vi "GE 5565PIORC.DMA.Block.In-Place Read (DBL).vi"(7 "count (-1: all)":i32=-1, 8 "error in (no error)":errorcluster, 9 "data in":dbl[](array[numeric]), 10 "Block Descriptor in":T1 {"descriptor params"."data ptr (lower)" format="%.0x"; "descriptor params"."data ptr (upper)" format="%.0x"; "descriptor params"."data size" format="%.0x"; "descriptor params"."next descriptor ptr" format="%.0x"; "descriptor size" format="%08x"; "descriptor ptr (RFM)" format="%08x"; "descriptor ptr (VISA)" format="%08x"}, 11 "GE 5565PIORC in":refnum<class "GE 5565PIORC.lvclass">) -> (0 "error out":errorcluster, 1 "data out":dbl[](array[numeric]), 2 "Block Descriptor out":T1 {"descriptor params"."data ptr (lower)" format="%.0x"; "descriptor params"."data ptr (upper)" format="%.0x"; "descriptor params"."data size" format="%.0x"; "descriptor params"."next descriptor ptr" format="%.0x"; "descriptor size" format="%08x"; "descriptor ptr (RFM)" format="%08x"; "descriptor ptr (VISA)" format="%08x"}, 3 "GE 5565PIORC out":refnum<class "GE 5565PIORC.lvclass">)   [LabVIEW 2016, in "GE 5565PIORC.lvclass"]
doc: "Reads <B>count</B> elements from the provided <B>Block Descriptor</B> into the provided <B>data</B> array. The number of elements transferred will be either <B>count</B> or the number of elements in <B>data</B>, whichever is smaller."
uses:
  GE 5565PIORC.lvclass
  Typedefs/GE 5565PIORC.Typedef.DMA Block Descriptor.ctl
  Typedefs/GE 5565PIORC.Typedef.DMA Block Descriptor Params.ctl
  GE 5565PIORC.lvclass/GE 5565PIORC.ctl
  <vilib>/Instr/_visa.llb/VISA Register Access Address Space.ctl
  GE 5565PIORC.VISA.Return Handler.vi
  <vilib>/Utility/error.llb/Error Cluster From Error Code.vi
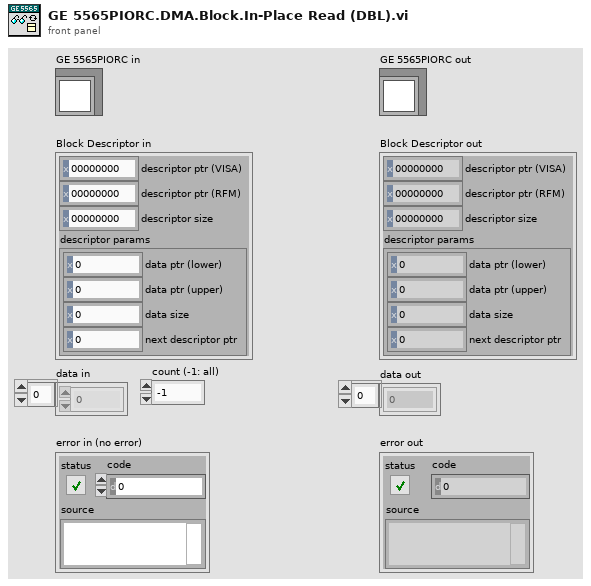
[diagram p1: front panel]
types:
  T1 = typedef "GE 5565PIORC.lvclass/GE 5565PIORC.Typedef.DMA Block Descriptor.ctl" = cluster{"descriptor ptr (VISA)":u32, "descriptor ptr (RFM)":u32, "descriptor size":u32, "descriptor params":T2}
  T2 = typedef "GE 5565PIORC.lvclass/GE 5565PIORC.Typedef.DMA Block Descriptor Params.ctl" = cluster{"data ptr (lower)":u32, "data ptr (upper)":u32, "data size":u32, "next descriptor ptr":u32}
  T3 = typedef "VISA Register Access Address Space.ctl" = u16
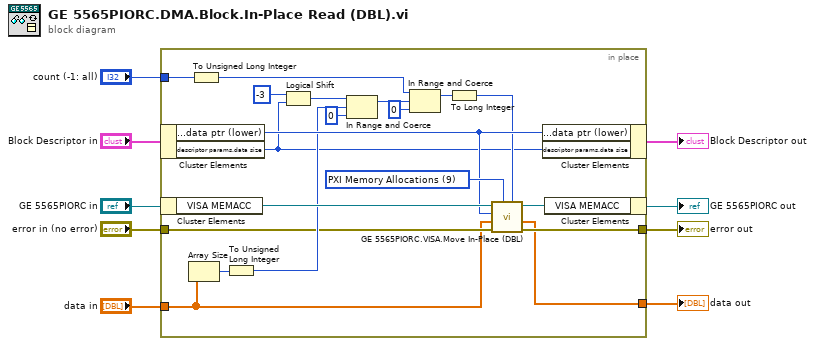
[diagram p0: block diagram]
diagram:
  n1 = in-place {
    in-place-border: "error in (no error)" -> [w15]
    in-place-border: [w27] -> w8
    in-place-border: [w21] -> w3
    in-place-border: "data in" -> [w10]
    in-place-border: "count (-1: all)" -> [w18]
    w25 = T3 9 items=["VXI/VME A16"=1, "VXI/VME A24"=2, "VXI/VME A32"=3, "VXI/VME A64"=4, "PXI Memory Allocations"=9, "PXI Configuration"=10, "PXI BAR0"=11, "PXI BAR1"=12, "PXI BAR2"=13, "PXI BAR3"=14, "PXI BAR4"=15, "PXI BAR5"=16] ("address space")
    n2 = in-place-cluster #1("Block Descriptor in") -> ("descriptor params.data ptr (lower)"=w24:u32, "descriptor params.data size"=w11:u32)
    n3 = in-place-cluster #2("GE 5565PIORC in") -> ("VISA MEMACC"=w26:refnum<visa-resource-name>)
    n4 = Array Size(array=w10) -> (size(s)=w20:i32)
    n5 = To Unsigned Long Integer(number=w18) -> (unsigned 32bit integer=w12:u32)
    n6 = To Unsigned Long Integer(number=w20) -> (unsigned 32bit integer=w19:u32)
    n7 = Logical Shift(y=i16 -3, x=w11) -> (x << y=w23:u32)
    n8 = In Range and Coerce(upper limit=w23, x=w19, lower limit=u32 0) -> (coerced(x)=w16:u32)  [unwired: 1 out]
    n9 = In Range and Coerce(upper limit=w12, x=w16, lower limit=u32 0) -> (coerced(x)=w14:u32)  [unwired: 1 out]
    n10 = To Long Integer(number=w14) -> (32bit integer=w13:i32)
    n11 = call "GE 5565PIORC.VISA.Move In-Place (DBL).vi"("count (-1: all)"=w13, "address space"=w25, "error in (no error)"=w15, "data in"=w10, "offset (0)"=w24, "VISA resource name"=w26) -> ("error out"=w27:errorcluster, "data out"=w21:dbl[], "VISA resource name out"=w28:refnum<visa-resource-name>)  [unwired: 3 in]
    n12 = in-place-cluster #1("descriptor params.data ptr (lower)"=w24, "descriptor params.data size"=w11) -> (→"Block Descriptor out":T1)
    n13 = in-place-cluster #2("VISA MEMACC"=w28) -> (→"GE 5565PIORC out":refnum<class "GE 5565PIORC.lvclass">)
  }
  "error out" <- w8
  "data out" <- w3
